vi "UpdateVIIcon.vi"(8 "error in (no error)":errorcluster, 10 "Method Name":string, 11 "VI in":refnum<vi>) -> (0 "error out":errorcluster, 3 "VI out":refnum<vi>)   [LabVIEW 2019, in "gRPC Template Creation Utility.lvlib"]
uses:
  gRPC Template Creation Utility.lvlib
  <vilib>/LabVIEW Icon API/API_Text.ctl
  <vilib>/LabVIEW Icon API/LabVIEW Icon API.lvlib
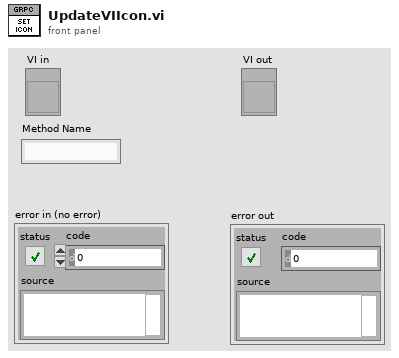
[diagram p1: front panel]
types:
  T1 = typedef "LabVIEW Icon API.lvlib/API_Text.ctl" = cluster{"Line 1 text":string, "Line 2 text":string, "Line 3 text":string, "Line 4 text":string}
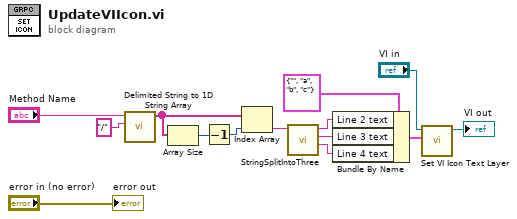
[diagram p0: block diagram]
diagram:
  n1 = call <vilib>:"Delimited String to 1D String Array.vi"("delimiter"="/", "delimited string"="Method Name") -> ("string array"=w4:string[])  [unwired: 9 in]
  n2 = Array Size(array=w4) -> (size(s)=w3:i32)
  n3 = Decrement(x=w3) -> (x-1=w2:i32)
  n4 = Index Array(array=w4, index=w2) -> (element=w1:string)
  n5 = call "StringSplitIntoThree.vi"("String"=w1) -> ("Line 3"=w7:string, "Line 2"=w8:string, "Line 1"=w9:string)  [unwired: 8 in]
  n6 = Bundle By Name(cluster=T1 {"Line 1 text"="", "Line 2 text"="a", "Line 3 text"="b", "Line 4 text"="c"} ("Text"), "Line 2 text"=w9, "Line 3 text"=w8, "Line 4 text"=w7) -> (w10:T1)
  n7 = call "Set VI Icon Text Layer.vi"("Text"=w10, "VI in"="VI in") -> ("VI out"=→"VI out":refnum<vi>)  [unwired: 8 in, 1 out]
  "error out" <- "error in (no error)"
